vi "niDTS WLAN INSTR TX Fetch Results.vi"(8 "error in (no error)":errorcluster, 10 "ActiveResultsSpace":u8=1, 11 "niDTS WLAN INSTR TX in":refnum<class "niDTS WLAN INSTR TX.lvclass">) -> (0 "error out":errorcluster, 2 "Resutls":T1 {"OBW"."Stop Frequency (Hz)" format="%#_4p"; "OBW"."Start Frequency (Hz)" format="%#_4p"; "OBW"."OBW (Hz)" format="%#_4p"}, 3 "niDTS WLAN INSTR TX out":refnum<class "niDTS WLAN INSTR TX.lvclass">)   [LabVIEW 2015, in "niDTS WLAN.lvlib" / "niDTS WLAN INSTR TX.lvclass"]
uses:
  niDTS WLAN INSTR TX.lvclass
  Tests/Tx Test/Includes/niDTS WLAN Tx Test INC Results.ctl
  Tests/Tx Test/Includes/niDTS WLAN Tx Test INC MOD EVM Results.ctl
  Tests/Tx Test/Includes/Results/niDTS Tx RES INC EVM.ctl
  Tests/Tx Test/Includes/niDTS WLAN Tx Test INC TXP Results.ctl
  Tests/Tx Test/Includes/niDTS WLAN Tx Test INC TXP Result SINGLE.ctl
  Tests/Tx Test/Includes/niDTS WLAN Tx Test INC OBW Results.ctl
  Results/niDTS WLAN INSTR TX INC SEM Results.ctl
  Results/niDTS WLAN INSTR TX INC SEM FSEGemts Results.ctl
  Tests/Tx Test/Includes/Results/niDTS Tx RES INC SEM FSEGemts.ctl
  Results/niDTS WLAN INSTR TX INC SEM MARGin Results.ctl
  Tests/Tx Test/Includes/Results/niDTS Tx RES INC SEM Margin.ctl
  Results/niDTS WLAN INSTR TX INC OFDM Impairments Results.ctl
  niDTS WLAN.lvlib
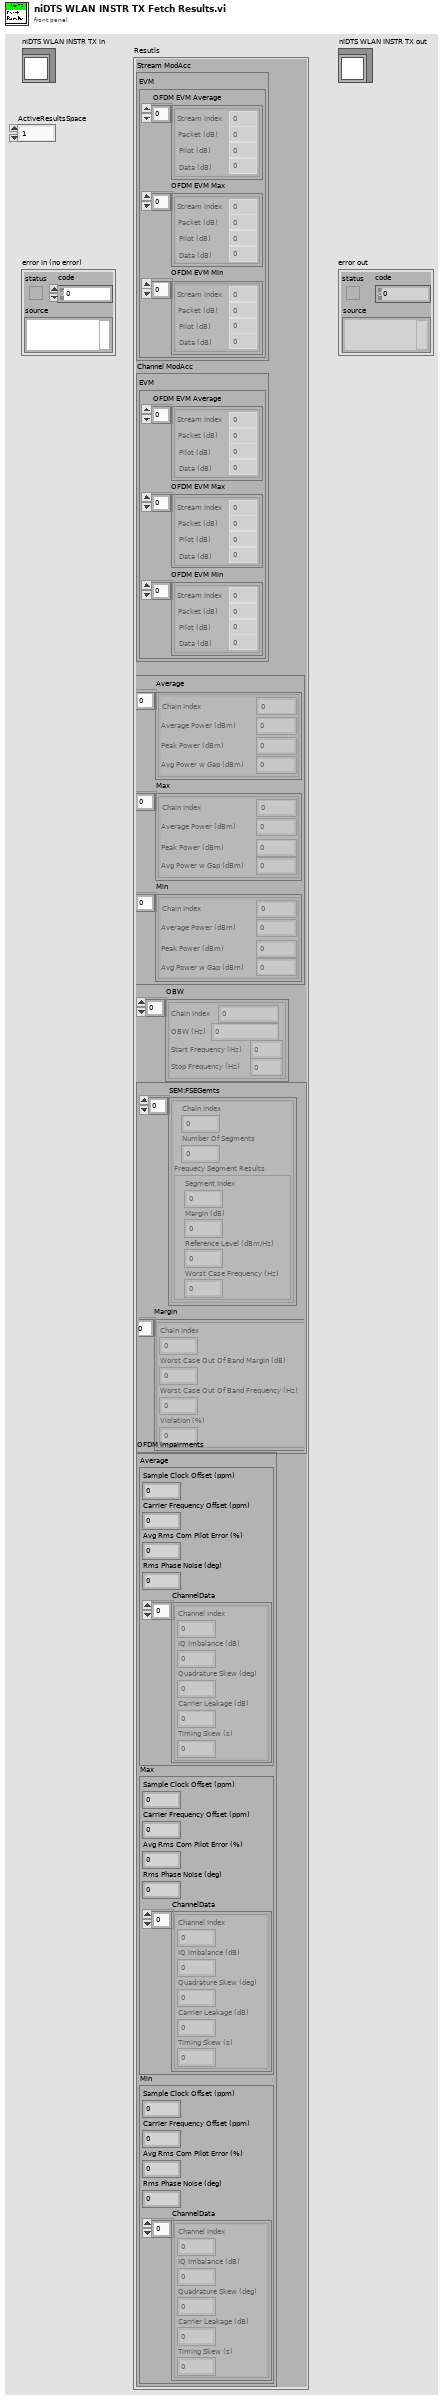
[diagram p1: front panel]
types:
  T1 = typedef "niDTS WLAN.lvlib/niDTS WLAN Tx Test INC Results.ctl" = cluster{"Stream ModAcc":T2, "Channel ModAcc":T2, "TXP":T4, "OBW":T6[], "SEM Results":T7, "OFDM Impairments":T12}
  T2 = typedef "niDTS WLAN.lvlib/niDTS WLAN Tx Test INC MOD EVM Results.ctl" = cluster{"EVM":cluster{"OFDM EVM Average":T3[], "OFDM EVM Max":T3[], "OFDM EVM Min":T3[]}}
  T3 = typedef "niDTS WLAN.lvlib/niDTS Tx RES INC EVM.ctl" = cluster{"Stream Index":i32, "Packet (dB)":dbl, "Pilot (dB)":dbl, "Data (dB)":dbl}
  T4 = typedef "niDTS WLAN.lvlib/niDTS WLAN Tx Test INC TXP Results.ctl" = cluster{"Average":T5[], "Max":T5[], "Min":T5[]}
  T5 = typedef "niDTS WLAN.lvlib/niDTS WLAN Tx Test INC TXP Result SINGLE.ctl" = cluster{"Chain Index":dbl, "Average Power (dBm)":dbl, "Peak Power (dBm)":dbl, "Avg Power w Gap (dBm)":dbl}
  T6 = typedef "niDTS WLAN.lvlib/niDTS WLAN Tx Test INC OBW Results.ctl" = cluster{"Chain Index":dbl, "OBW (Hz)":dbl, "Start Frequency (Hz)":dbl, "Stop Frequency (Hz)":dbl}
  T7 = typedef "niDTS WLAN.lvlib/niDTS WLAN INSTR TX.lvclass/niDTS WLAN INSTR TX INC SEM Results.ctl" = cluster{"SEM:FSEGemts":T8, "Margin":T10}
  T8 = typedef "niDTS WLAN.lvlib/niDTS WLAN INSTR TX.lvclass/niDTS WLAN INSTR TX INC SEM FSEGemts Results.ctl" = T9[]
  T9 = typedef "niDTS WLAN.lvlib/niDTS Tx RES INC SEM FSEGemts.ctl" = cluster{"Chain Index":i32, "Number Of Segments":i32, "Frequecy Segment Results":cluster{"Segment Index":i32, "Margin (dB)":dbl, "Reference Level (dBm/Hz)":dbl, "Worst Case Frequency (Hz)":dbl}}
  T10 = typedef "niDTS WLAN.lvlib/niDTS WLAN INSTR TX.lvclass/niDTS WLAN INSTR TX INC SEM MARGin Results.ctl" = T11[]
  T11 = typedef "niDTS WLAN.lvlib/niDTS Tx RES INC SEM Margin.ctl" = cluster{"Chain Index":i32, "Worst Case Out Of Band Margin (dB)":dbl, "Worst Case Out Of Band Frequency (Hz)":dbl, "Violation (%)":dbl}
  T12 = typedef "niDTS WLAN.lvlib/niDTS WLAN INSTR TX.lvclass/niDTS WLAN INSTR TX INC OFDM Impairments Results.ctl" = cluster{"Average":cluster{"Sample Clock Offset (ppm)":dbl, "Carrier Frequency Offset (ppm)":dbl, "Avg Rms Com Pilot Error (%)":dbl, "Rms Phase Noise (deg)":dbl, "ChannelData":cluster{"Channel Index":i32, "IQ Imbalance (dB)":dbl, "Quadrature Skew (deg)":dbl, "Carrier Leakage (dB)":dbl, "Timing Skew (s)":dbl}[]}, "Max":cluster{"Sample Clock Offset (ppm)":dbl, "Carrier Frequency Offset (ppm)":dbl, "Avg Rms Com Pilot Error (%)":dbl, "Rms Phase Noise (deg)":dbl, "ChannelData":cluster{"Channel Index":i32, "IQ Imbalance (dB)":dbl, "Quadrature Skew (deg)":dbl, "Carrier Leakage (dB)":dbl, "Timing Skew (s)":dbl}[]}, "Min":cluster{"Sample Clock Offset (ppm)":dbl, "Carrier Frequency Offset (ppm)":dbl, "Avg Rms Com Pilot Error (%)":dbl, "Rms Phase Noise (deg)":dbl, "ChannelData":cluster{"Channel Index":i32, "IQ Imbalance (dB)":dbl, "Quadrature Skew (deg)":dbl, "Carrier Leakage (dB)":dbl, "Timing Skew (s)":dbl}[]}}
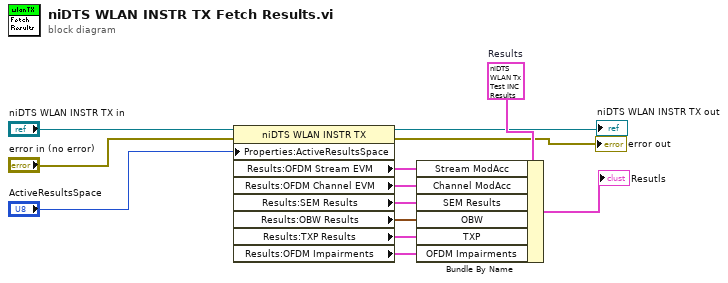
[diagram p0: block diagram]
diagram:
  w12 = T1 {"Stream ModAcc"={"EVM"={"OFDM EVM Average"=[], "OFDM EVM Max"=[], "OFDM EVM Min"=[]}}, "Channel ModAcc"={"EVM"={"OFDM EVM Average"=[], "OFDM EVM Max"=[], "OFDM EVM Min"=[]}}, "TXP"={"Average"=[], "Max"=[], "Min"=[]}, "OBW"=[], "SEM Results"={"SEM:FSEGemts"=[], "Margin"=[]}, "OFDM Impairments"={"Average"={"Sample Clock Offset (ppm)"=0.0, "Carrier Frequency Offset (ppm)"=0.0, "Avg Rms Com Pilot Error (%)"=0.0, "Rms Phase Noise (deg)"=0.0, "ChannelData"=[]}, "Max"={"Sample Clock Offset (ppm)"=0.0, "Carrier Frequency Offset (ppm)"=0.0, "Avg Rms Com Pilot Error (%)"=0.0, "Rms Phase Noise (deg)"=0.0, "ChannelData"=[]}, "Min"={"Sample Clock Offset (ppm)"=0.0, "Carrier Frequency Offset (ppm)"=0.0, "Avg Rms Com Pilot Error (%)"=0.0, "Rms Phase Noise (deg)"=0.0, "ChannelData"=[]}}}  # Results
  n1 = property class="niDTS WLAN INSTR TX"(reference="niDTS WLAN INSTR TX in", error in="error in (no error)", "Properties:ActiveResultsSpace"="ActiveResultsSpace") -> (reference out=→"niDTS WLAN INSTR TX out":refnum<class "niDTS WLAN INSTR TX.lvclass">, error out=→"error out":errorcluster, "Results:OFDM Stream EVM"=w2:T2, "Results:OFDM Channel EVM"=w7:T2, "Results:SEM Results"=w6:T7, "Results:OBW Results"=w5:T6[], "Results:TXP Results"=w4:T4, "Results:OFDM Impairments"=w3:T12)
  n2 = Bundle By Name(cluster=w12, "Stream ModAcc"=w2, "Channel ModAcc"=w7, "SEM Results"=w6, "OBW"=w5, "TXP"=w4, "OFDM Impairments"=w3) -> (→"Resutls":T1)
